vi "MultiOpto_1.3_Begin.vi"() -> (9 "NI DMM 3 option return":enum32{"Ampermeter button", "Ohmmeter button"}(ring), 11 "NI DMM 2 option return":enum32{"Ampermeter button", "Ohmmeter button"}(ring), 13 "NI DMM 1 option return":enum32{"Ampermeter button", "Ohmmeter button"}(ring), 15 "Stepper Motor Status":bool, 17 "Ophir 2 Status":bool, 18 "Текущий Образец №":string, 19 "Ophir 1 Status":bool, 20 "DC Power 1 Status":bool, 21 "DC Power 2 Status":bool, 22 "DC Power 3 Status":bool, 23 "DC Power 4 Status":bool, 24 "NI DMM 1 Status":bool, 25 "NI DMM 2 Status":bool, 26 "NI DMM 3 Status":bool, 27 "NI Scope Status":bool)   [LabVIEW 2018]
panel:
  in  "DC Power 4":bool
  in  "DC Power 3":bool
  in  "DC Power 1":bool
  in  "DC Power 2":bool
  in  "OK Button":bool
  in  "Stepper Motor":bool
  in  "NI DMM 3 option":enum32{"Ampermeter button", "Ohmmeter button"}(radio)
  in  "NI DMM 3":bool
  in  "NI DMM 2 option":enum32{"Ampermeter button", "Ohmmeter button"}(radio)
  in  "NI DMM 1 option":enum32{"Ampermeter button", "Ohmmeter button"}(radio)
  in  "Ophir 2":bool
  in  "NI DMM 2":bool
  out "Boolean 4":bool
  out "Boolean 3":bool
  in  "Ophir 1":bool
  in  "NI DMM 1":bool
  in  "NI Scope":bool
  in  "Образец №":string
  out "Boolean":bool
  out "Boolean 2":bool
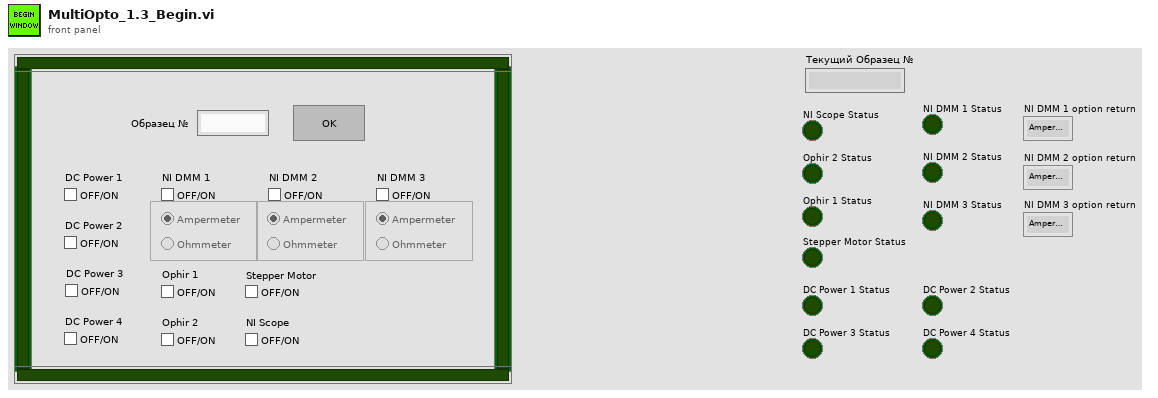
[diagram p1: front panel]
types:
  T1 = enum8{"Enabled", "Disabled", "Disabled and Grayed Out"}
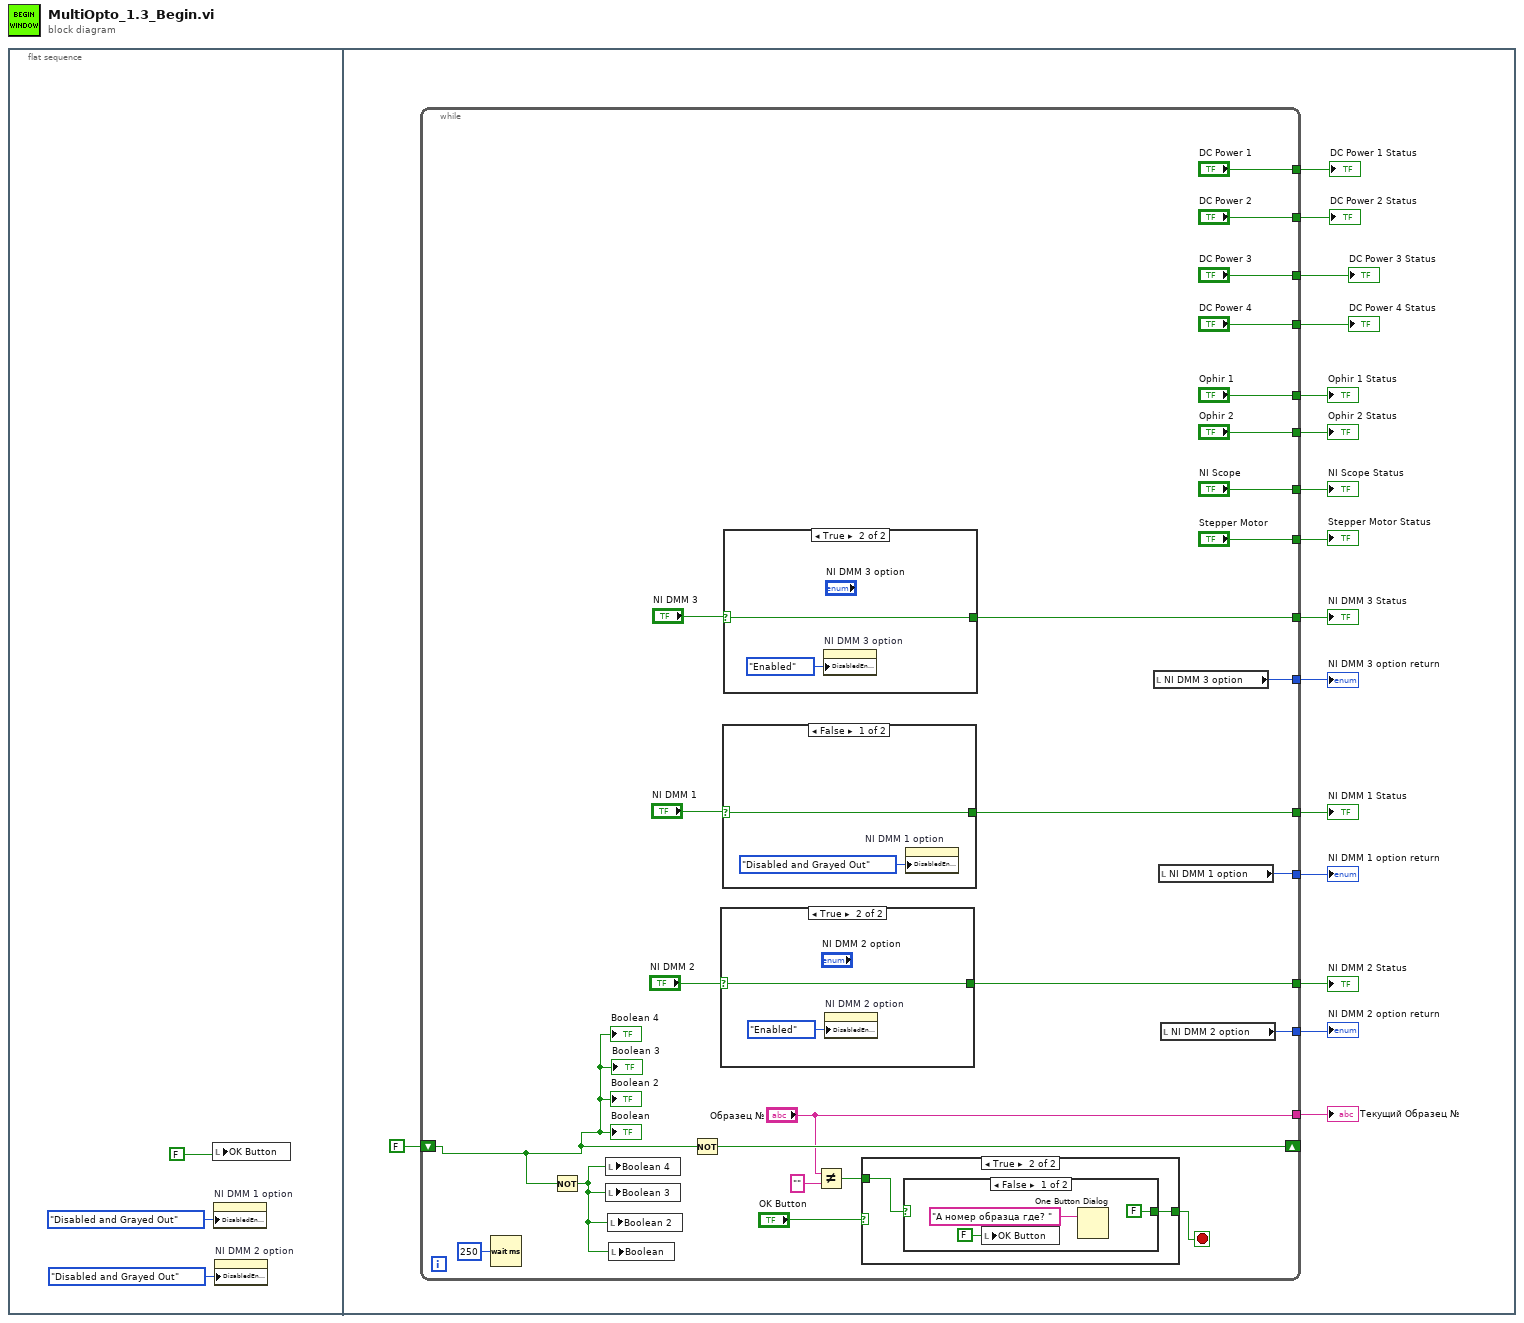
[diagram p0: block diagram]
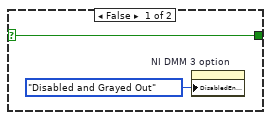
[diagram p4: hidden frame]
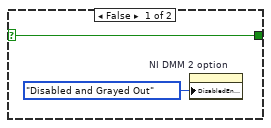
[diagram p5: hidden frame]
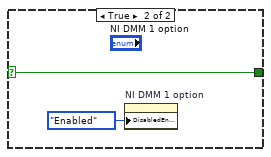
[diagram p6: hidden frame]
diagram:
  n1 = flat-sequence {
    frame #0 {
      n2 = local write "OK Button"(FALSE ("Ввел!")) -> ()
      n3 = property on="NI DMM 1 option" class="RadioBtnsControl (strict)"("DisabledEnum"=T1."Disabled and Grayed Out" ("Disabled")) -> ()  [unwired: 2 in, 2 out]
      n4 = property on="NI DMM 2 option" class="RadioBtnsControl (strict)"("DisabledEnum"=T1."Disabled and Grayed Out" ("Disabled")) -> ()  [unwired: 2 in, 2 out]
    }
    frame #1 {
      n5 = while {
        tunnel: ["Образец №"] -> w19
        shift-right: [w44] -> _
        shift-left: FALSE -> [w43]
        tunnel: ["NI Scope"] -> w17
        tunnel: [w36] -> w16
        tunnel: ["Ophir 1"] -> w15
        tunnel: [w35] -> w14
        tunnel: ["Ophir 2"] -> w13
        tunnel: [w34] -> w12
        tunnel: [w33] -> w11
        tunnel: [w31] -> w10
        tunnel: [w30] -> w9
        tunnel: ["Stepper Motor"] -> w8
        tunnel: ["DC Power 1"] -> w7
        tunnel: ["DC Power 2"] -> w6
        tunnel: ["DC Power 3"] -> w5
        tunnel: ["DC Power 4"] -> w4
        stop <- w26 stop-if-true
        n6 = Wait (ms)(milliseconds to wait=u32 250) -> ()  [unwired: 1 out]
        n7 = Not(x=w43) -> (.not. x?=w42:bool)
        n8 = local write "Boolean 4"(w42) -> ()
        n9 = local write "Boolean 3"(w42) -> ()
        n10 = local write "Boolean 2"(w42) -> ()
        n11 = local write "Boolean"(w42) -> ()
        n12 = Not(x=w43) -> (.not. x?=w44:bool)
        n13 = case shown="True" "NI DMM 2" {
          selector: "NI DMM 2" -> [w57 w60]
          tunnel: [w57 w60] -> w35
          frame False {
            n14 = property on="NI DMM 2 option" class="RadioBtnsControl (strict)"("DisabledEnum"=T1."Disabled and Grayed Out" ("Disabled")) -> ()  [unwired: 2 in, 2 out]
          }
          frame True {
            n15 = property on="NI DMM 2 option" class="RadioBtnsControl (strict)"("DisabledEnum"=T1."Enabled" ("Disabled")) -> ()  [unwired: 2 in, 2 out]
          }
        }
        n16 = case shown="False" "NI DMM 1" {
          selector: "NI DMM 1" -> [w61 w64]
          tunnel: [w61 w64] -> w36
          frame False {
            n17 = property on="NI DMM 1 option" class="RadioBtnsControl (strict)"("DisabledEnum"=T1."Disabled and Grayed Out" ("Disabled")) -> ()  [unwired: 2 in, 2 out]
          }
          frame True {
            n18 = property on="NI DMM 1 option" class="RadioBtnsControl (strict)"("DisabledEnum"=T1."Enabled" ("Disabled")) -> ()  [unwired: 2 in, 2 out]
          }
        }
        n19 = case shown="True" "NI DMM 3" {
          selector: "NI DMM 3" -> [w53 w56]
          tunnel: [w53 w56] -> w31
          frame False {
            n20 = property on="NI DMM 3 option" class="RadioBtnsControl (strict)"("DisabledEnum"=T1."Disabled and Grayed Out" ("Disabled")) -> ()  [unwired: 2 in, 2 out]
          }
          frame True {
            n21 = property on="NI DMM 3 option" class="RadioBtnsControl (strict)"("DisabledEnum"=T1."Enabled" ("Disabled")) -> ()  [unwired: 2 in, 2 out]
          }
        }
        n22 = Not Equal?(x="Образец №", y="") -> (x != y?=w27:bool)
        n23 = case shown="True" "OK Button" {
          selector: "OK Button" -> [w46 _]
          tunnel: w27 -> [_ w48]
          tunnel: [w46 w47] -> w26
          frame False {
          }
          frame True {
            n24 = case shown="False" w48 {
              selector: w48 -> [_ w52]
              tunnel: [FALSE w52] -> w47
              frame False {
                n25 = local write "OK Button"(FALSE ("OK Button")) -> ()
                n26 = One Button Dialog(message="А номер образца где? ") -> ()  [unwired: 1 in, 1 out]
              }
              frame True {
              }
            }
          }
        }
        n27 = local read "NI DMM 3 option"() -> (w30:enum32{"Ampermeter button", "Ohmmeter button"})
        n28 = local read "NI DMM 1 option"() -> (w34:enum32{"Ampermeter button", "Ohmmeter button"})
        n29 = local read "NI DMM 2 option"() -> (w33:enum32{"Ampermeter button", "Ohmmeter button"})
        "Boolean" <- w43
        "Boolean 2" <- w43
        "Boolean 3" <- w43
        "Boolean 4" <- w43
      }
      "Текущий Образец №" <- w19
      "NI Scope Status" <- w17
      "NI DMM 1 Status" <- w16
      "Ophir 1 Status" <- w15
      "NI DMM 2 Status" <- w14
      "Ophir 2 Status" <- w13
      "NI DMM 2 option return" <- w11
      "NI DMM 1 option return" <- w12
      "NI DMM 3 Status" <- w10
      "NI DMM 3 option return" <- w9
      "Stepper Motor Status" <- w8
      "DC Power 1 Status" <- w7
      "DC Power 2 Status" <- w6
      "DC Power 3 Status" <- w5
      "DC Power 4 Status" <- w4
    }
  }
